vi "Record Continuous Tags Rev 170821_A.vi"(0 "Run Letter":string="a", 1 "path":path=path "C:/Fuel Lab Bench Testing/Test Data/Oil Pump 171121", 2 "Waveform Array In":waveform(dbl)[](array[waveform]), 4 "Force Record":bool caption="Force Record Enable", 6 "Main Count":dbl, 7 "Num_Blocks":dbl=13.0, 9 "Record Disable":bool caption="Record Enable", 10 "Data Tag":dbl format="%.2p", 11 "Record \"Num_Blocks\"":bool=TRUE caption="Disable") -> (3 "Record Cmd":bool, 5 "Recorded Blocks":dbl, 8 "Saving Data":bool)   [LabVIEW 2017]
uses:
  <vilib>/ptbypt/NI_PtbyPt.lvlib
panel:
  out "Main Count 2":dbl
  out "x .or. y?":bool
  in  "Data In":dbl
  out "Data Out":dbl
  in  "direction":enum16{"either", "false-true", "true-false"}(ring)=enum."false-true"
  # "Rev 131203_A, added \".lvm\" file extension to file path.\nRev 141029 adds block counter to allow fixed number of blocks recorded.\nRev 151208_A records to TDMS file type instead of the text-based \".lvm\".   This can be changed inside the \"Write to Measurement File.vi\" Express VI.\nRev 160128_A changes logic so that Force Record can override Data Tag # critieria.\nRev 161209_A prepends \"\\\" to filename so that the new file goes inside the desired directory.  This is being used initially in the Fuel Lab.\nRev 161212_A outputs number of blocks logged."
  # "N:\\TeamShares\\Testing Group\\Bench Tests\\PR19321 - Cooler Pressure Drop - Orthrus\\Valve PD"
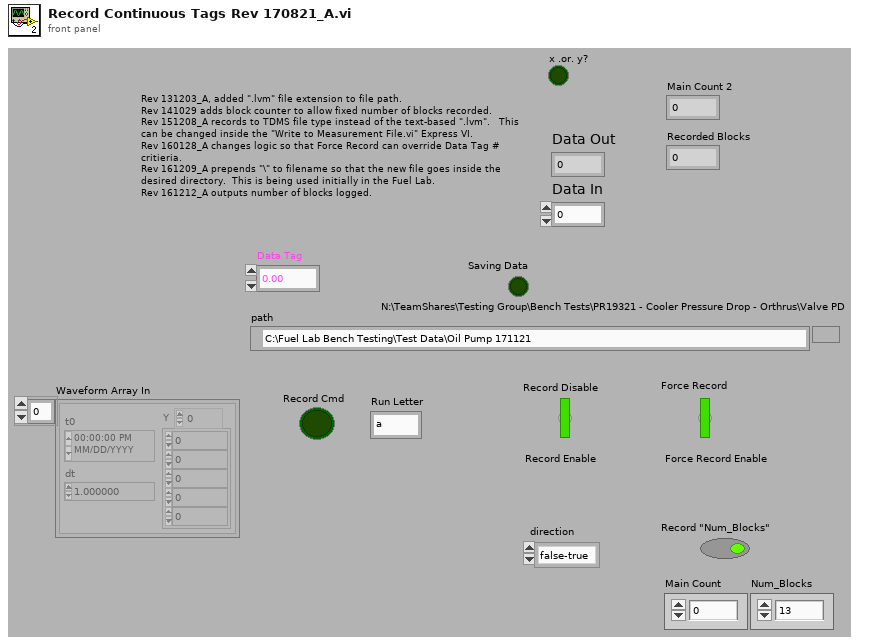
[diagram p1: front panel]
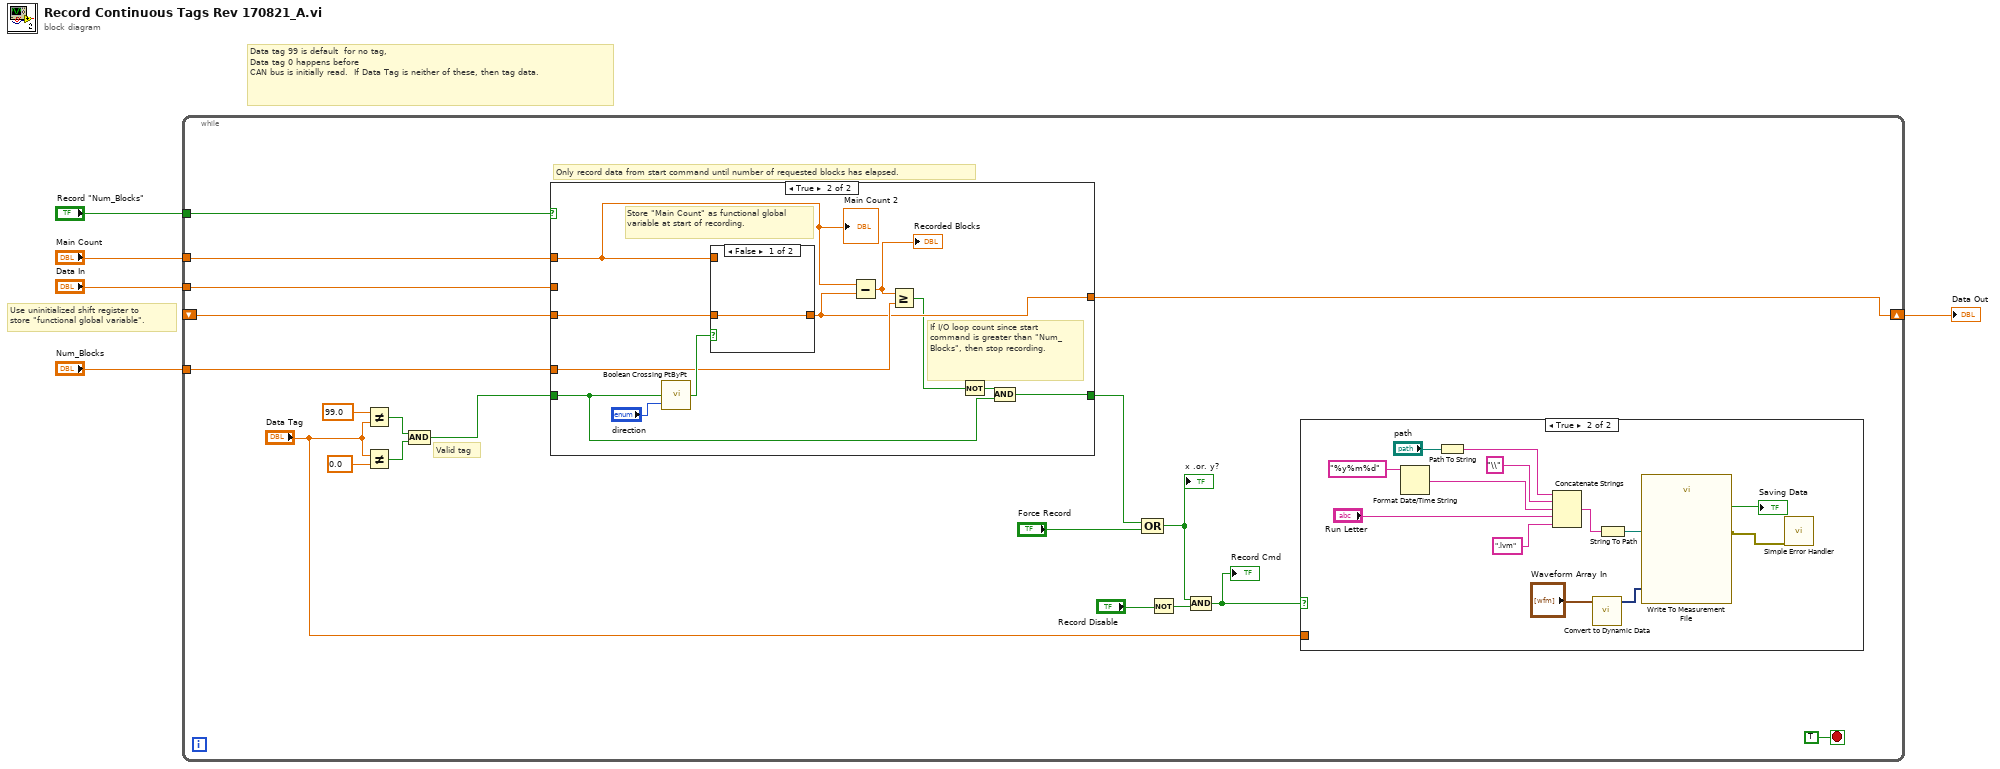
[diagram p0: block diagram]
diagram:
  # "Use uninitialized shift register to store \"functional global variable\"."
  # "Data tag 99 is default  for no tag,\nData tag 0 happens before \nCAN bus is initially read.  If Data Tag is neither of these, then tag data."
  n1 = while {
    shift-right: [w9] -> w3
    shift-left: _ -> [w12]
    tunnel: "Main Count" -> [w11]
    tunnel: "Record \"Num_Blocks\"" -> [w10]
    tunnel: "Data In" -> [w8]
    tunnel: "Num_Blocks" -> [w7]
    stop <- TRUE stop-if-true
    # "Valid tag"
    # "Only record data from start command until number of requested blocks has elapsed."
    n2 = Not Equal?(x=99.0 ("y"), y="Data Tag") -> (x != y?=w16:bool)
    n3 = Not Equal?(x="Data Tag", y=0.0 ("x")) -> (x != y?=w18:bool)
    n4 = And(x=w16, y=w18) -> (x .and. y?=w15:bool)
    n5 = case shown="True" w10 {
      tunnel: w15 -> [w39 w42]
      tunnel: [w39 w43] -> w21
      tunnel: w11 -> [_ w48]
      tunnel: w7 -> [_ w47]
      tunnel: w12 -> [_ w45]
      tunnel: [w38 w44] -> w9
      tunnel: w8 -> [w38 _]
      frame False {
      }
      frame True {
        # "If I/O loop count since start command is greater than \"Num_Blocks\", then stop recording."
        # "Store \"Main Count\" as functional global variable at start of recording."
        n6 = call <vilib>:"Boolean Crossing PtByPt.vi"("direction"="direction", "input"=w42) -> ("crossing"=w49:bool)  [unwired: 1 in]
        n7 = case shown="False" w49 {
          tunnel: w48 -> [_ w52]
          tunnel: [w51 w52] -> w44
          tunnel: w45 -> [w51 _]
          frame False {
          }
          frame True {
          }
        }
        n8 = Subtract(x=w48, y=w44) -> (x-y=w46:dbl)
        "Recorded Blocks" <- w46
        n9 = Greater Or Equal?(x=w46, y=w47) -> (x >= y?=w40:bool)
        n10 = Not(x=w40) -> (.not. x?=w41:bool)
        n11 = And(x=w41, y=w42) -> (x .and. y?=w43:bool)
        "Main Count 2" <- w48
      }
    }
    n12 = Compound Arithmetic op=OR(w21, "Force Record") -> (w22:bool)
    "x .or. y?" <- w22
    n13 = Not(x="Record Disable") -> (.not. x?=w23:bool)
    n14 = And(x=w22, y=w23) -> (x .and. y?=w20:bool)
    "Record Cmd" <- w20
    n15 = case shown="True" w20 {
      tunnel: "Data Tag" -> [_ _]
      frame False {
      }
      frame True {
        n16 = Format Date/Time String(time format string (%c)="%y%m%d" ("string")) -> (date/time string=w34:string)  [unwired: 2 out]
        n17 = Path To String(path="path") -> (string=w27:string)
        n18 = Concatenate Strings(w27, "\\" ("string"), w34, "Run Letter", ".lvm" ("string")) -> (w33:string)
        n19 = call "Convert to Dynamic Data"("Array of Waveforms"="Waveform Array In") -> ("Dynamic Data Type"=w31:dynamicdata)  [unwired: 3 in]
        n20 = String To Path(string=w33) -> (path=w30:path)
        n21 = call "Write To Measurement File"("Signals"=w31, "Filename"=w30) -> ("Saving Data"=→"Saving Data":bool, "error out"=w29:errorcluster)  [unwired: 15 in, 1 out]
        n22 = call <vilib>:"Simple Error Handler.vi"("error in (no error)"=w29) -> ()  [unwired: 1 in, 8 out]
      }
    }
  }
  "Data Out" <- w3
